vi "Write All Child Attributes.vi"(10 "All Child Attributes":T1, 11 "TEMPLATE Actor in":refnum<class "TEMPLATE Actor.lvclass">) -> (3 "TEMPLATE Actor out":refnum<class "TEMPLATE Actor.lvclass">)   [LabVIEW 2025, in "_Template.lvlib" / "Templates.lvlib" / "TEMPLATE Actor.lvlib" / "TEMPLATE Actor.lvlib" / "TEMPLATE Actor.lvclass"]
uses:
  TEMPLATE Actor.lvclass
  jettl/jettl/All Child Attributes.ctl
  jettl/jettl/Attributes/Attributes.lvclass
  TEMPLATE Actor.lvclass/TEMPLATE Actor.ctl
  C:/git/jettl/src/jettl Tools/_Template/Templates/TEMPLATE Actor/TEMPLATE Actor/TEMPLATE Actor/TEMPLATE Actor.lvclass
  C:/git/jettl/src/jettl/jettl/Actor/Actor.lvclass
  jettl/jettl/jettl.lvlib
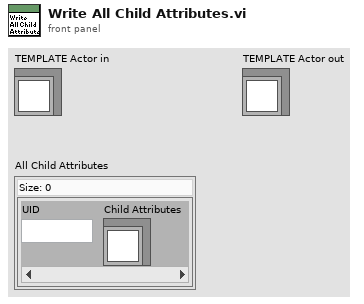
[diagram p1: front panel]
types:
  T1 = typedef "jettl.lvlib/All Child Attributes.ctl" = map{string, refnum<class "Attributes.lvclass">}
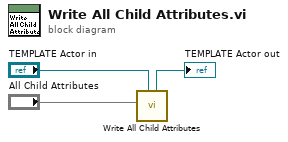
[diagram p0: block diagram]
diagram:
  n1 = call "Write All Child Attributes.vi"("Actor in"="TEMPLATE Actor in", "All Child Attributes"="All Child Attributes") -> ("Actor out"=→"TEMPLATE Actor out":refnum<class "TEMPLATE Actor.lvclass">)  [unwired: 9 in]
